vi "TLB Native Dynamic Events ver 0.04b beta.vi"() -> ()   [LabVIEW 2018]
uses:
  Labview Training Phase 2/Enum Controls/States for Action Engine.ctl
  Type def/TLB event states.ctl
  Type def/TLB MHL States.ctl
panel:
  out "Action Queue Items":i32
  out "State Logic Queue Items":i32
  out "Action Queues items":string[](array[string])=["Hardware reset", "Software reset", ""]
  out "State logic":T1=enum."Task 2"
  out "Action State":string
  in  "Task Execution Mode":bool
  in  "Tasks Selector":string(combo)="Task 2"
  in  "Stop Queue":bool
  in  "Start Task":bool
  # "Test Programme written by Calvin Loke    Dated: 28 Aug 2019\nTest Programme revised by Dr Alex See   Dated 30 Aug 2019\n\nProgramme version:   TLB Native Dynamic Events ver 0.04b.vi"
  # "System Health Status Update"
  # "Sequence of Actions"
  # "Continuous (Repeated)"
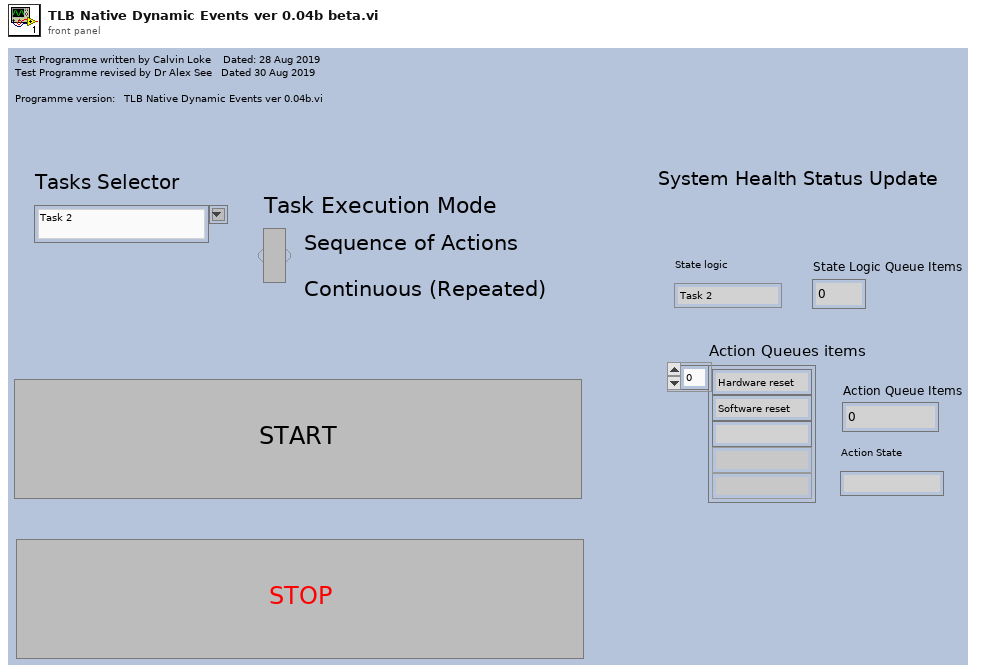
[diagram p1: front panel]
types:
  T1 = typedef "TLB MHL States.ctl" = enum16{"None", "Startup", "Idle", "Processing", "Shutdown", "Reset", "Task 1", "Task 2", "Task 3", "Task 4", "Task 4a", "Task 4b", "Task 4c", "Task 4d", "Task 4e", "Task 4f", "Task 4g", "Task 4h", "Acquire image", "Wall follow mode", "Autodrive", "Autodrive a"}
  T2 = typedef "States for Action Engine.ctl" = enum16{"Initialize", "Write", "Read"}
  T3 = typedef "TLB event states.ctl" = enum16{"Start Sequence", "Exit", "Start Task 1", "Start Task 2", "Start Task 3", "Start Task 4", "Camera vision", "Wall follow mode", "Idle", "Start Drive Straight"}
  T4 = typedef "TLB event states.ctl" = enum16{"Start Sequence", "Exit", "Task 1", "Task 2", "Idle"}
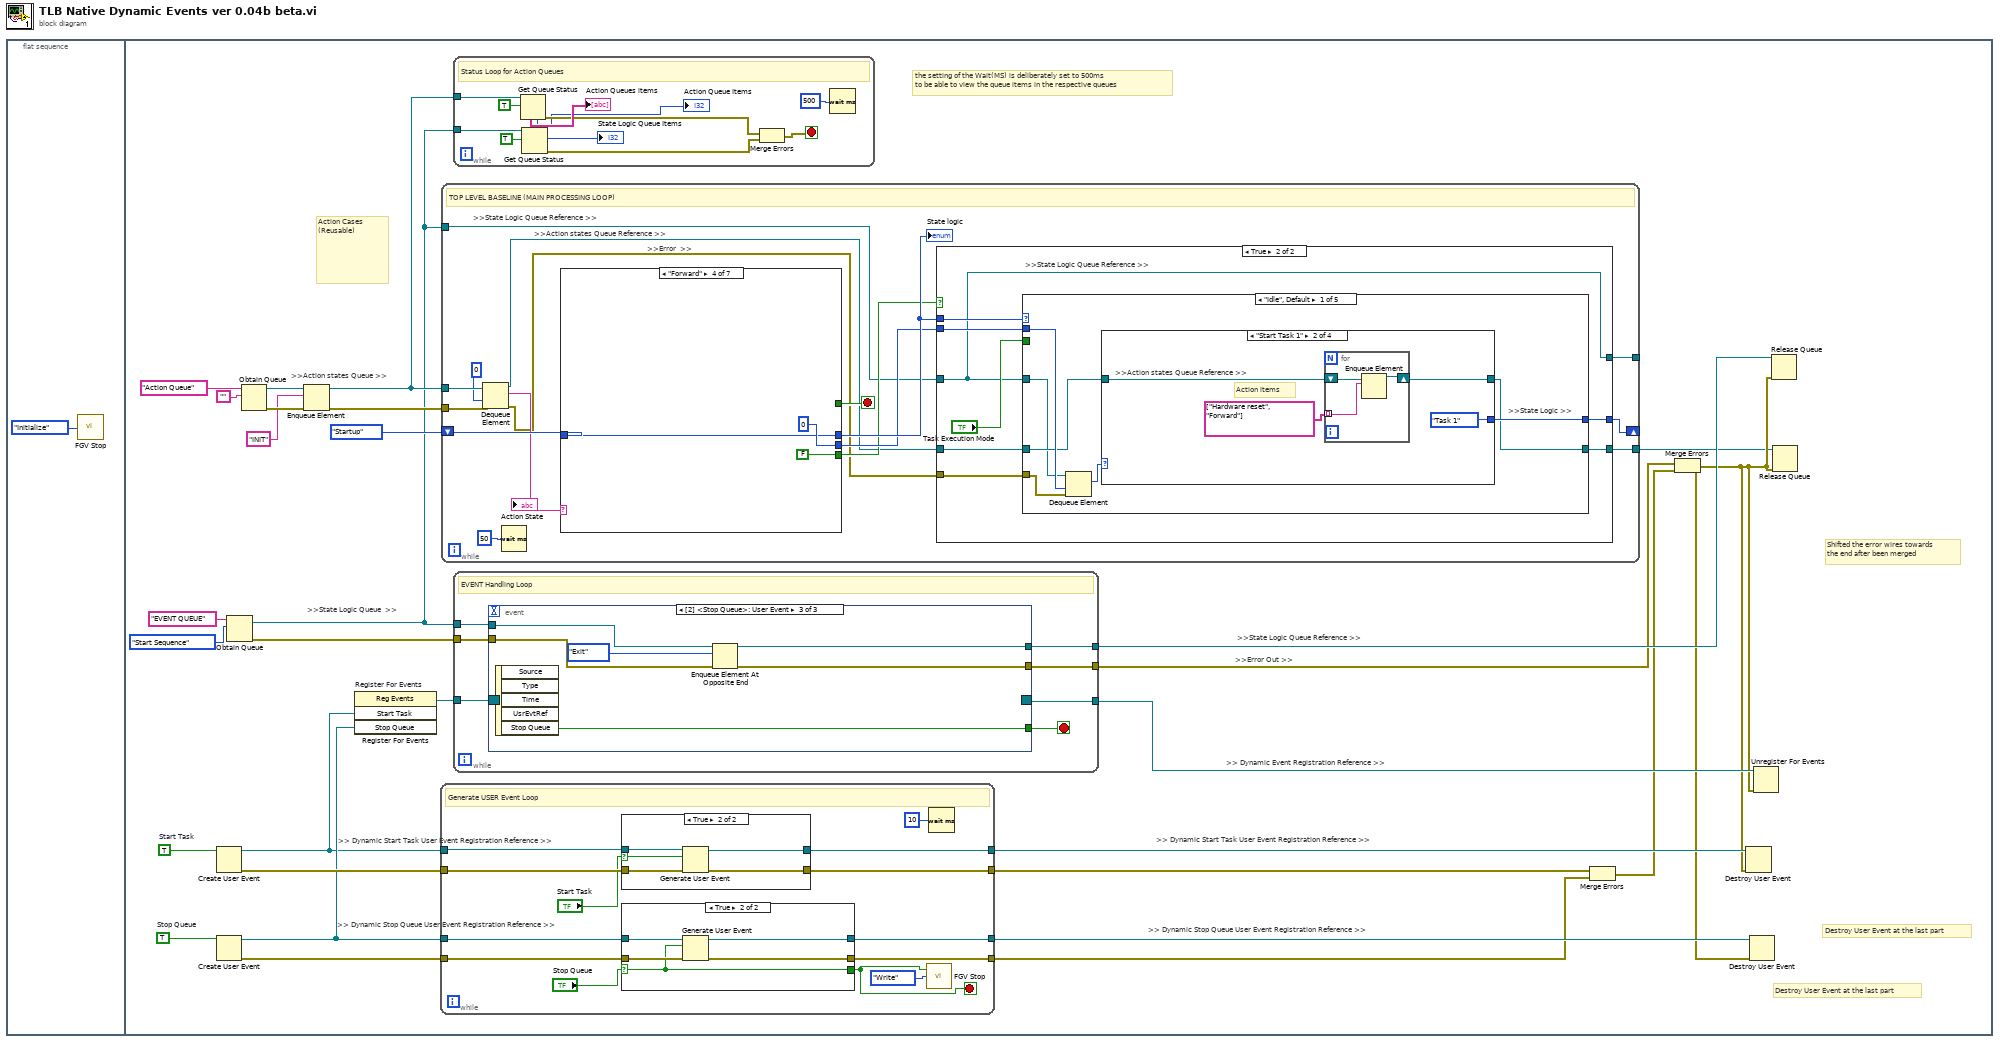
[diagram p0: block diagram]
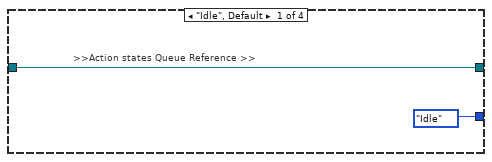
[diagram p3: hidden frame]
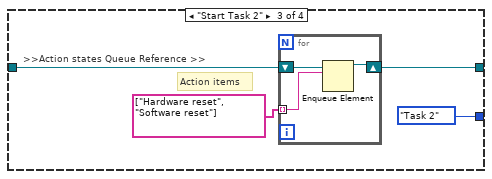
[diagram p4: hidden frame]
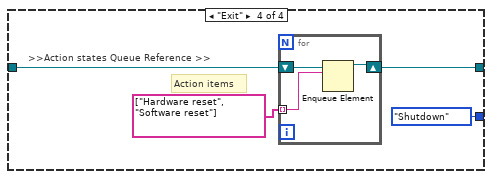
[diagram p5: hidden frame]
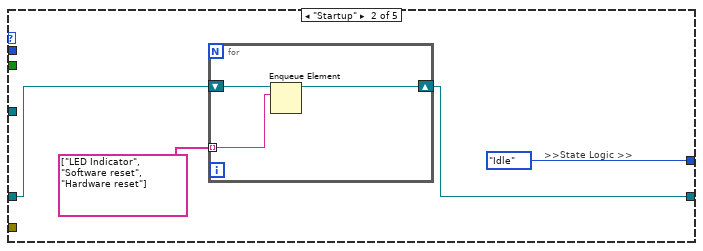
[diagram p6: hidden frame]
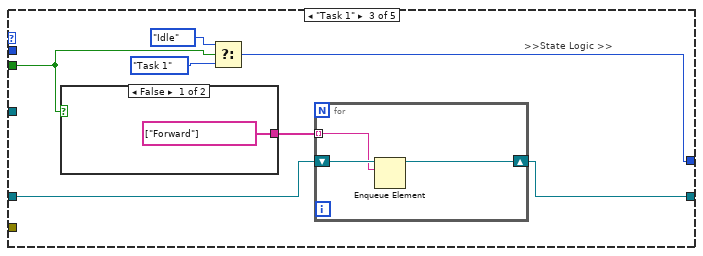
[diagram p7: hidden frame]
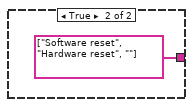
[diagram p8: hidden frame]
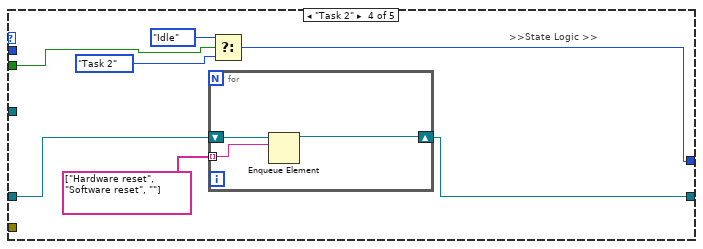
[diagram p9: hidden frame]
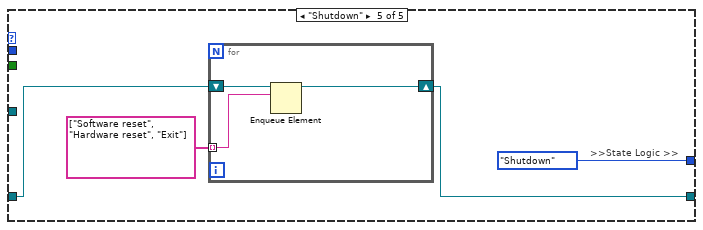
[diagram p10: hidden frame]
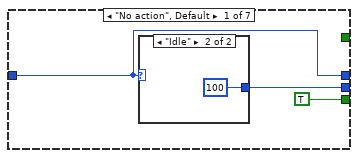
[diagram p11: hidden frame]
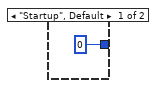
[diagram p12: hidden frame]
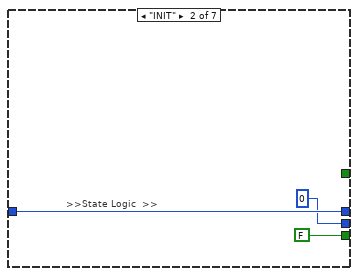
[diagram p13: hidden frame]
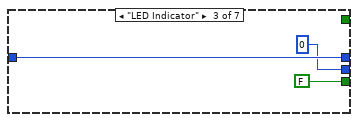
[diagram p14: hidden frame]
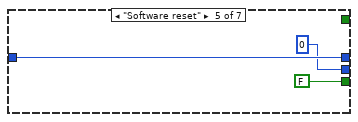
[diagram p15: hidden frame]
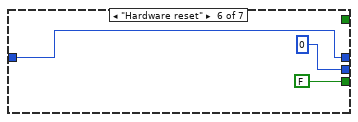
[diagram p16: hidden frame]
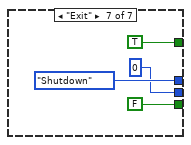
[diagram p17: hidden frame]
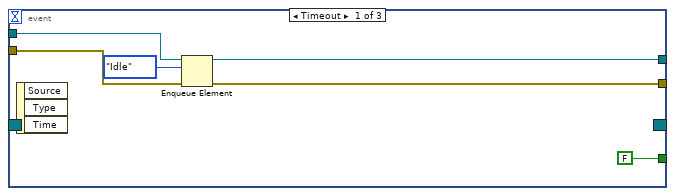
[diagram p18: hidden frame]
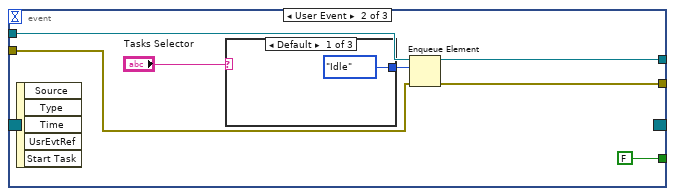
[diagram p19: hidden frame]
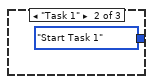
[diagram p20: hidden frame]
diagram:
  n1 = flat-sequence {
    frame #0 {
      n2 = call "FGV Stop.vi"("Init/Read/Write State"=States_for_Action_Engine."Initialize") -> ()  [unwired: 2 in, 2 out]
    }
    frame #1 {
      w30 = TRUE  # Stop Queue
      w29 = TRUE  # Start Task
      # "the setting of the Wait(MS) is deliberately set to 500ms\nto be able to view the queue items in the respective queues"
      # "Action Cases\n(Reusable)"
      # ">>Error Out >>"
      # ">> Dynamic Stop Queue User Event Registration Reference >>"
      # ">> Dynamic Start Task User Event Registration Reference >>"
      # ">> Dynamic Stop Queue User Event Registration Reference >>"
      # ">> Dynamic Start Task User Event Registration Reference >>"
      # ">> Dynamic Event Registration Reference >>"
      # ">>Action states Queue >>"
      # ">>State Logic Queue  >>"
      # ">>State Logic Queue Reference >>"
      # "Destroy User Event at the last part"
      # "Destroy User Event at the last part"
      # "Shifted the error wires towards\nthe end after been merged"
      n3 = Create User Event(user event datatype=w29) -> (user event=w21:refnum<user-event>, error out=w26:errorcluster)  [unwired: 1 in]
      n4 = Create User Event(user event datatype=w30) -> (user event=w22:refnum<user-event>, error out=w25:errorcluster)  [unwired: 1 in]
      n5 = Obtain Queue(name (unnamed)="EVENT QUEUE", element data type=TLB_event_states."Start Sequence" ("Enum")) -> (queue out=w5:refnum<queue>, error out=w11:errorcluster)  [unwired: 3 in, 1 out]
      n6 = Obtain Queue(name (unnamed)="Action Queue", element data type="") -> (queue out=w14:refnum<queue>, error out=w10:errorcluster)  [unwired: 3 in, 1 out]
      n7 = Enqueue Element(queue=w14, element="INIT", error in (no error)=w10) -> (queue out=w6:refnum<queue>, error out=w9:errorcluster)  [unwired: 1 in, 1 out]
      n8 = register-events "Register For Events"(w21, w22) -> (reference out=w20:refnum<event-registration>)  [unwired: 2 in, 1 out]
      n9 = while {
        tunnel: w21 -> [w199]
        tunnel: w22 -> [w198]
        tunnel: [w197] -> w28
        tunnel: [w196] -> w27
        tunnel: w26 -> [w195]
        tunnel: [w194] -> w24
        tunnel: w25 -> [w193]
        tunnel: [w192] -> w23
        stop <- w188 stop-if-true
        # "Generate USER Event Loop"
        n10 = case shown="True" "Start Task" {
          selector: "Start Task" -> [_ w211]
          tunnel: w199 -> [w210 w215]
          tunnel: [w210 w214] -> w196
          tunnel: w195 -> [w209 w213]
          tunnel: [w209 w212] -> w194
          frame False {
          }
          frame True {
            n11 = Generate User Event(user event=w215, event data cluster=w211, error in=w213) -> (user event out=w214:refnum<user-event>, error out=w212:errorcluster)  [unwired: 1 in]
          }
        }
        n12 = case shown="True" "Stop Queue" {
          selector: "Stop Queue" -> [_ w204]
          tunnel: w198 -> [w203 w208]
          tunnel: [w203 w207] -> w197
          tunnel: w193 -> [w202 w206]
          tunnel: [w202 w205] -> w192
          tunnel: [FALSE w204] -> w188
          frame False {
          }
          frame True {
            n13 = Generate User Event(user event=w208, event data cluster=w204, error in=w206) -> (user event out=w207:refnum<user-event>, error out=w205:errorcluster)  [unwired: 1 in]
          }
        }
        n14 = call "FGV Stop.vi"("Init/Read/Write State"=States_for_Action_Engine."Write", "Input Node"=w188) -> ()  [unwired: 1 in, 2 out]
        n15 = Wait (ms)(milliseconds to wait=u32 10) -> ()  [unwired: 1 out]
      }
      n16 = while {
        tunnel: w5 -> [w44]
        shift-right: [w49] -> _
        shift-left: TLB_MHL_States."Startup" ("Enum") -> [w56]
        tunnel: w6 -> [w54]
        tunnel: w9 -> [w52]
        tunnel: [w51] -> _
        tunnel: [w50] -> w3
        stop <- w47 stop-if-true
        # ">>Error  >>"
        # ">>Action states Queue Reference >>"
        # ">>State Logic Queue Reference >>"
        # "TOP LEVEL BASELINE (MAIN PROCESSING LOOP)"
        n17 = Dequeue Element(queue=w54, timeout in ms (-1)=0, error in (no error)=w52) -> (queue out=w43:refnum<queue>, element=w53:string, error out=w42:errorcluster)  [unwired: 1 out]
        "Action State" <- w53
        n18 = Wait (ms)(milliseconds to wait=u32 50) -> ()  [unwired: 1 out]
        n19 = case shown="\"Forward\"" w53 {
          tunnel: [w137 w142 w145 w147 w151 w154 TLB_MHL_States."Shutdown" ("Enum")] -> w55
          tunnel: w56 -> [w137 w142 w145 w147 w151 w154 _]
          tunnel: [w136 0 0 0 0 0 0] -> w48
          tunnel: [_ _ _ _ _ _ TRUE] -> w47
          tunnel: [TRUE FALSE FALSE FALSE FALSE FALSE FALSE] -> w46
          frame "No action", Default {
            n20 = case shown="\"Idle\"" w137 {
              tunnel: [0 100] -> w136
              frame "Startup", Default {
              }
              frame "Idle" {
              }
            }
          }
          frame "INIT" {
            # ">>State Logic  >>"
          }
          frame "LED Indicator" {
          }
          frame "Forward" {
          }
          frame "Software reset" {
          }
          frame "Hardware reset" {
          }
          frame "Exit" {
          }
        }
        "State logic" <- w55
        n21 = case shown="True" w46 {
          tunnel: w55 -> [w59 w68]
          tunnel: w44 -> [w60 w61]
          tunnel: w43 -> [w58 w67]
          tunnel: [w60 w61] -> w51
          tunnel: [w58 w66] -> w50
          tunnel: [w59 w65] -> w49
          tunnel: w42 -> [_ w64]
          tunnel: w48 -> [_ w63]
          frame False {
          }
          frame True {
            # ">>State Logic Queue Reference >>"
            n22 = case shown="\"Idle\", Default" w68 {
              tunnel: w61 -> [w69 _ _ _ _]
              tunnel: w67 -> [w71 w100 w107 w119 w129]
              tunnel: [w70 w99 w106 w120 w128] -> w66
              tunnel: [w74 TLB_MHL_States."Idle" ("Enum") w110 w122 TLB_MHL_States."Shutdown" ("Enum")] -> w65
              tunnel: w64 -> [w72 _ _ _ _]
              tunnel: w63 -> [w73 _ _ _ _]
              tunnel: "Task Execution Mode" -> [_ _ w109 w118 _]
              frame "Idle", Default {
                # ">>State Logic >>"
                n23 = Dequeue Element(queue=w69, timeout in ms (-1)=w73, error in (no error)=w72) -> (element=w75:T3)  [unwired: 3 out]
                n24 = case shown="\"Start Task 1\"" w75 {
                  tunnel: [TLB_MHL_States."Idle" ("Enum") TLB_MHL_States."Task 1" ("Enum") TLB_MHL_States."Task 2" ("Enum") TLB_MHL_States."Shutdown" ("Enum")] -> w74
                  tunnel: [w76 w80 w85 w92] -> w70
                  tunnel: w71 -> [w76 w78 w86 w93]
                  frame "Idle", Default {
                    # ">>Action states Queue Reference >>"
                  }
                  frame "Start Task 1" {
                    # ">>Action states Queue Reference >>"
                    # "Action items"
                    n25 = for {
                      shift-right: [w84] -> w80
                      shift-left: w78 -> [w83]
                      tunnel: string[] ["Hardware reset", "Forward"] -> [w82] mode=indexing
                      n26 = Enqueue Element(queue=w83, element=w82) -> (queue out=w84:refnum<queue>)  [unwired: 2 in, 2 out]
                    }
                  }
                  frame "Start Task 2" {
                    # ">>Action states Queue Reference >>"
                    # "Action items"
                    n27 = for {
                      shift-right: [w91] -> w85
                      shift-left: w86 -> [w90]
                      tunnel: string[] ["Hardware reset", "Software reset"] -> [w89] mode=indexing
                      n28 = Enqueue Element(queue=w90, element=w89) -> (queue out=w91:refnum<queue>)  [unwired: 2 in, 2 out]
                    }
                  }
                  frame "Exit" {
                    # ">>Action states Queue Reference >>"
                    # "Action items"
                    n29 = for {
                      shift-right: [w98] -> w92
                      shift-left: w93 -> [w97]
                      tunnel: string[] ["Hardware reset", "Software reset"] -> [w96] mode=indexing
                      n30 = Enqueue Element(queue=w97, element=w96) -> (queue out=w98:refnum<queue>)  [unwired: 2 in, 2 out]
                    }
                  }
                }
              }
              frame "Startup" {
                # ">>State Logic >>"
                n31 = for {
                  shift-right: [w104] -> w99
                  shift-left: w100 -> [w105]
                  tunnel: string[] ["LED Indicator", "Software reset", "Hardware reset"] -> [w103] mode=indexing
                  n32 = Enqueue Element(queue=w105, element=w103) -> (queue out=w104:refnum<queue>)  [unwired: 2 in, 2 out]
                }
              }
              frame "Task 1" {
                # ">>State Logic >>"
                n33 = case shown="False" w109 {
                  tunnel: [string[] ["Forward"] string[] ["Software reset", "Hardware reset", ""]] -> w108
                  frame False {
                  }
                  frame True {
                  }
                }
                n34 = Select(t=TLB_MHL_States."Idle" ("Enum"), s=w109, f=TLB_MHL_States."Task 1" ("Enum")) -> (s? t:f=w110:T1)
                n35 = for {
                  shift-right: [w116] -> w106
                  shift-left: w107 -> [w117]
                  tunnel: w108 -> [w115] mode=indexing
                  n36 = Enqueue Element(queue=w117, element=w115) -> (queue out=w116:refnum<queue>)  [unwired: 2 in, 2 out]
                }
              }
              frame "Task 2" {
                # ">>State Logic >>"
                n37 = for {
                  shift-right: [w126] -> w120
                  shift-left: w119 -> [w127]
                  tunnel: string[] ["Hardware reset", "Software reset", ""] -> [w125] mode=indexing
                  n38 = Enqueue Element(queue=w127, element=w125) -> (queue out=w126:refnum<queue>)  [unwired: 2 in, 2 out]
                }
                n39 = Select(t=TLB_MHL_States."Idle" ("Enum"), s=w118, f=TLB_MHL_States."Task 2" ("Enum")) -> (s? t:f=w122:T1)
              }
              frame "Shutdown" {
                # ">>State Logic >>"
                n40 = for {
                  shift-right: [w133] -> w128
                  shift-left: w129 -> [w134]
                  tunnel: string[] ["Software reset", "Hardware reset", "Exit"] -> [w132] mode=indexing
                  n41 = Enqueue Element(queue=w134, element=w132) -> (queue out=w133:refnum<queue>)  [unwired: 2 in, 2 out]
                }
              }
            }
          }
        }
      }
      n42 = while {
        tunnel: w6 -> [w39]
        tunnel: w5 -> [w36]
        stop <- w33 stop-if-true
        # "Status Loop for Action Queues"
        n43 = Get Queue Status(queue=w39, return elements? (F)=TRUE) -> (error out=w35:errorcluster, # elements in queue=→"Action Queue Items":i32, elements=→"Action Queues items":string[])  [unwired: 1 in, 5 out]
        n44 = Get Queue Status(queue=w36, return elements? (F)=TRUE) -> (# pending remove=→"State Logic Queue Items":i32, error out=w34:errorcluster)  [unwired: 1 in, 6 out]
        n45 = Merge Errors(w35, w34) -> (w33:errorcluster)
        n46 = Wait (ms)(milliseconds to wait=u32 500) -> ()  [unwired: 1 out]
      }
      n47 = while {
        tunnel: w20 -> [w165]
        tunnel: [w164] -> w19
        tunnel: w5 -> [w162]
        tunnel: [w161] -> w18
        tunnel: w11 -> [w160]
        tunnel: [w159] -> w8
        stop <- w163 stop-if-true
        # "EVENT Handling Loop"
        n48 = event shown="[2] <Stop Queue>: User Event" {
          selector: w165 -> [_ _ _]
          dyn-events: [_ _ _] -> w164
          timeout: _ -> [_ _ _]
          tunnel: [FALSE FALSE w187] -> w163
          tunnel: w162 -> [w170 w177 w185]
          tunnel: [w169 w176 w186] -> w161
          tunnel: w160 -> [w167 w173 w183]
          tunnel: [w166 w172 w182] -> w159
          event Timeout {
            n49 = event-data() -> ()  [unwired: 1 in, 3 out]
            n50 = Enqueue Element(queue=w170, element=TLB_event_states."Idle" ("Enum"), error in (no error)=w167) -> (queue out=w169:refnum<queue>, error out=w166:errorcluster)  [unwired: 1 in, 1 out]
          }
          event User Event {
            n51 = event-data() -> ()  [unwired: 1 in, 5 out]
            n52 = case shown="Default" "Tasks Selector" {
              tunnel: [TLB_event_states."Idle" ("Enum") TLB_event_states."Start Task 1" ("Enum") TLB_event_states."Task 2" ("Enum")] -> w174
              frame Default {
              }
              frame "Task 1" {
              }
              frame "Task 2" {
              }
            }
            n53 = Enqueue Element(queue=w177, element=w174, error in (no error)=w173) -> (queue out=w176:refnum<queue>, error out=w172:errorcluster)  [unwired: 1 in, 1 out]
          }
          event User Event {
            n54 = event-data() -> ("Stop Queue"=w187:bool)  [unwired: 1 in, 4 out]
            n55 = Enqueue Element At Opposite End(queue=w185, element=TLB_event_states."Exit" ("Enum"), error in (no error)=w183) -> (queue out=w186:refnum<queue>, error out=w182:errorcluster)  [unwired: 1 in, 1 out]
          }
        }
      }
      n56 = Merge Errors "Merge Errors"(w24, w23) -> (w2:errorcluster)
      n57 = Merge Errors(w8, w2) -> (w4:errorcluster)
      n58 = Destroy User Event(user event=w27, error in=w4) -> ()  [unwired: 1 out]
      n59 = Destroy User Event(user event=w28, error in=w4) -> ()  [unwired: 1 out]
      n60 = Unregister For Events(event registration refnum=w19, error in=w4) -> ()  [unwired: 1 out]
      n61 = Release Queue(queue=w18, error in (no error)=w4) -> ()  [unwired: 1 in, 3 out]
      n62 = Release Queue(queue=w3, error in (no error)=w4) -> ()  [unwired: 1 in, 3 out]
    }
  }
